vi "read.volume.map.vi"(8 "error in":errorcluster, 11 "volume index filepath":path=path "D:/Comics/data/key_maps/volumes.json") -> (0 "error out":errorcluster, 3 "volume_map":T1(array[cluster]))   [LabVIEW 2024]
uses:
  definitions/volume.index--cluster.ctl
  <vilib>/addons/_JKI.lib/Serialization/JSON/JKI JSON Serialization.lvlib
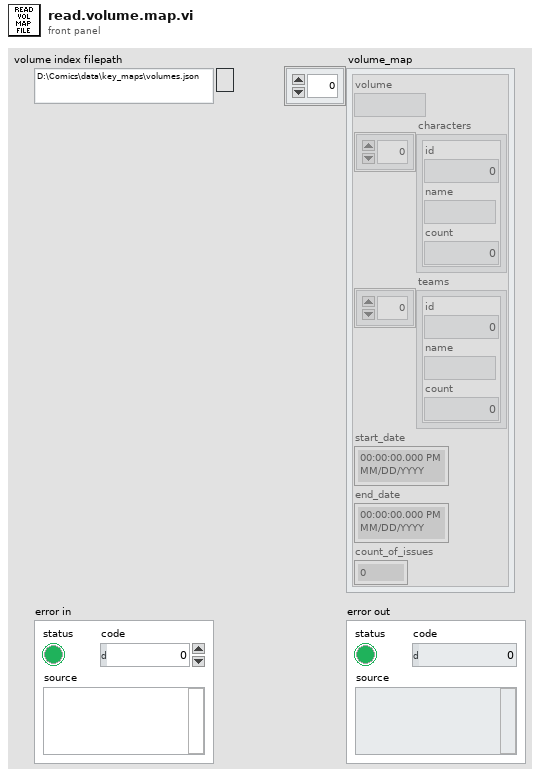
[diagram p1: front panel]
types:
  T1 = cluster{"volume":string, "characters":cluster{"id":i32, "name":string, "count":i32}[], "teams":cluster{"id":i32, "name":string, "count":i32}[], "start_date":timestamp, "end_date":timestamp, "count_of_issues":i32}[]
  T2 = typedef "volume.index--cluster.ctl" = cluster{"volume_map":cluster{"volume":string, "characters":cluster{"id":i32, "name":string, "count":i32}[], "teams":cluster{"id":i32, "name":string, "count":i32}[], "start_date":timestamp, "end_date":timestamp, "count_of_issues":i32}[]}
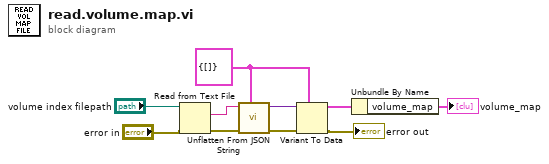
[diagram p0: block diagram]
diagram:
  w5 = T2 {"volume_map"=[]} ("volume index")
  n1 = Read from Text File(file (use dialog)="volume index filepath", error in="error in") -> (text=w8:string, error out=w9:errorcluster)  [unwired: 2 in, 2 out]
  n2 = call <vilib>:"Unflatten From JSON String.vi"("Type and Defaults"=w5, "error in"=w9, "JSON String"=w8) -> ("error out"=w7:errorcluster, "Variant"=w6:variant)  [unwired: 7 in]
  n3 = Variant To Data(error in=w7, type=w5, Variant=w6) -> (data=w4:T2, error out=→"error out":errorcluster)
  n4 = Unbundle By Name(w4) -> ("volume_map"=→"volume_map":T1)
